vi "Feedback Message Loop.vi"(8 "error in (no error)":errorcluster, 10 "Data Notifiers":T2, 11 "Message Queues":T6) -> (0 "error out":errorcluster)   [LabVIEW 2013, in "Feedback.lvlib"]
uses:
  Feedback.lvlib
  support/Message Queue/All Message Queues.ctl
  support/Message Queue/Message Cluster.ctl
  Feedback State.ctl
  Feedback Parameters.ctl
  Scan Parameters.ctl
  support/Data Notifiers/All Data Notifiers.ctl
  Acquisition/APD Notifier Cluster.ctl
  Piezo/Piezo display.ctl
  XY/XY Display.ctl
  Capacitive/Capacitive Signal Cluster.ctl
  Error Signal.ctl
  piezo new/Hardware Configuration Piezo.ctl
  <vilib>/Utility/error.llb/Error Cluster From Error Code.vi
  support/Message Queue/Enqueue Message (Single).vi
  <vilib>/ErrorRing/Error Ring.xnode
  support/Message Queue/Message Queue.lvlib
  Piezo/Piezo.lvlib
  Acquisition/Acquisition.lvlib
  XY/XY.lvlib
  support/Data Notifiers/Data Notifiers.lvlib
  Capacitive/Capacitive.lvlib
panel:
  in  "Feedback Settings 2":T1={"Setpoint (cnt)"=3.0, "Refresh Time (s)"=1.0, "K_p (nm/cnt)"=0.01, "Averaging Time"=1.0, "T_i (s)"=1.0, "T_d (s)"=0.0, "Error Signal Source"=0} {"Error Signal Source" items=["External Input", "APD Signal"]}
  in  "Feedback Settings":T1={"Setpoint (cnt)"=3.0, "Refresh Time (s)"=1.0, "K_p (nm/cnt)"=0.01, "Averaging Time"=1.0, "T_i (s)"=1.0, "T_d (s)"=0.0, "Error Signal Source"=0} {"Error Signal Source" items=["External Input", "APD Signal"]}
  out "running average":dbl[](graph)
  out "Feedback State":T3 {"Feedback Parameters"."Error Signal Source" items=["External Input", "APD Signal"]}
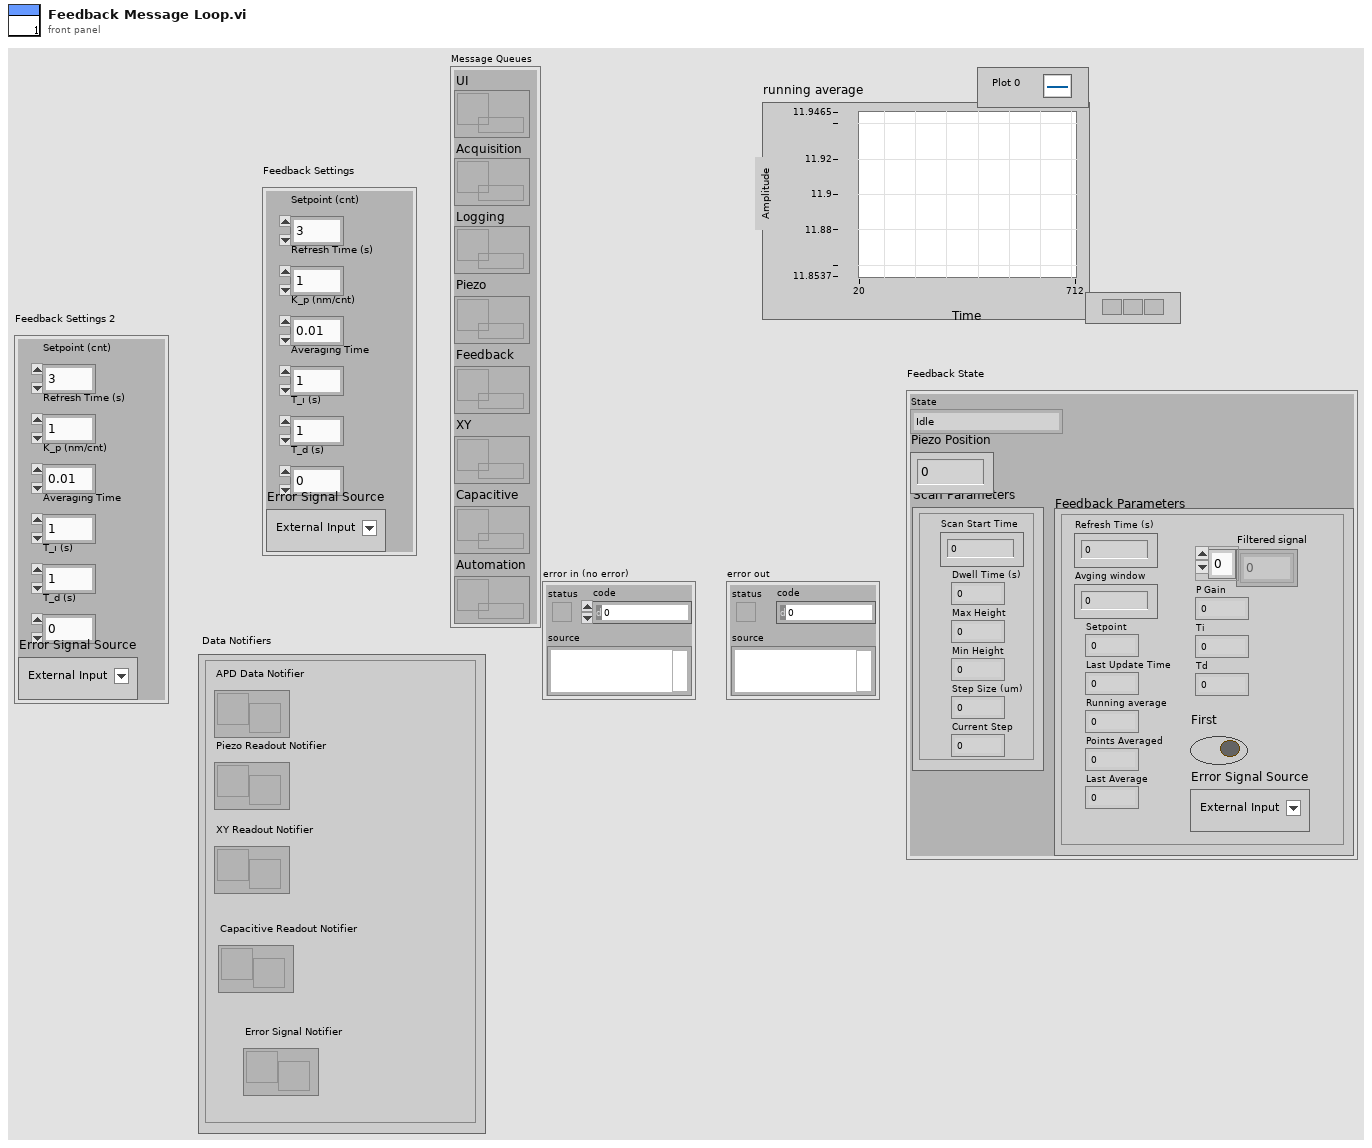
[diagram p1: front panel]
types:
  T1 = cluster{"Setpoint (cnt)":dbl, "Refresh Time (s)":dbl, "K_p (nm/cnt)":dbl, "Averaging Time":dbl, "T_i (s)":dbl, "T_d (s)":dbl, "Error Signal Source":u16}
  T2 = typedef "Data Notifiers.lvlib/All Data Notifiers.ctl" = cluster{"APD Data Notifier":refnum<notifier>, "Piezo Readout Notifier":refnum<notifier>, "XY Readout Notifier":refnum<notifier>, "Capacitive Readout Notifier":refnum<notifier>, "Error Signal Notifier":refnum<notifier>}
  T3 = typedef "Feedback.lvlib/Feedback State.ctl" = cluster{"State":enum16{"Idle", "Feedback", "Scanning", "Averaging"}, "Feedback Parameters":T4, "Scan Parameters":T5, "Piezo Position":dbl}
  T4 = typedef "Feedback.lvlib/Feedback Parameters.ctl" = cluster{"Refresh Time (s)":dbl, "P Gain":dbl, "Setpoint":dbl, "Last Update Time":dbl, "Running average":dbl, "Points Averaged":dbl, "Last Average":dbl, "Filtered signal":dbl[], "Avging window":dbl, "Ti":dbl, "Td":dbl, "First":bool, "Error Signal Source":u16}
  T5 = typedef "Feedback.lvlib/Scan Parameters.ctl" = cluster{"Scan Start Time":dbl, "Step Size (um)":dbl, "Min Height":dbl, "Max Height":dbl, "Dwell Time (s)":dbl, "Current Step":dbl}
  T6 = typedef "Message Queue.lvlib/All Message Queues.ctl" = cluster{"UI":refnum<queue>, "Acquisition":refnum<queue>, "Logging":refnum<queue>, "Piezo":refnum<queue>, "Feedback":refnum<queue>, "XY":refnum<queue>, "Capacitive":refnum<queue>, "Automation":refnum<queue>}
  T7 = typedef "Piezo.lvlib/Hardware Configuration Piezo.ctl" = cluster{"DAQmx Channel":tag, "Max Input":dbl, "Min Input":dbl, "Samples per ch.":dbl, "Setpoint (um)":dbl, "DAQmx Task":refnum<k21>}
  T8 = typedef "Feedback.lvlib/Error Signal.ctl" = cluster{"Error signal":dbl[], "Setpoint":dbl, "Last average":dbl}
  T9 = enum16{"Idle", "Feedback", "Scanning", "Averaging"}
  T10 = cluster{"Averaging Time (s)\n":dbl, "Error Signal Source":u16}
  T11 = cluster{"Dwell Time (s)":dbl, "Max Height":dbl, "Min Height":dbl, "Step Size (um)":dbl}
  T12 = typedef "Piezo.lvlib/Piezo display.ctl" = cluster{"PiezoPosition":sgl, "Counter Time":i32}
  T13 = typedef "Capacitive.lvlib/Capacitive Signal Cluster.ctl" = cluster{"Readout":sgl, "Time":i32, "Temperature":dbl}
  T14 = typedef "Acquisition.lvlib/APD Notifier Cluster.ctl" = cluster{"data":dbl[][], "t0":i32}
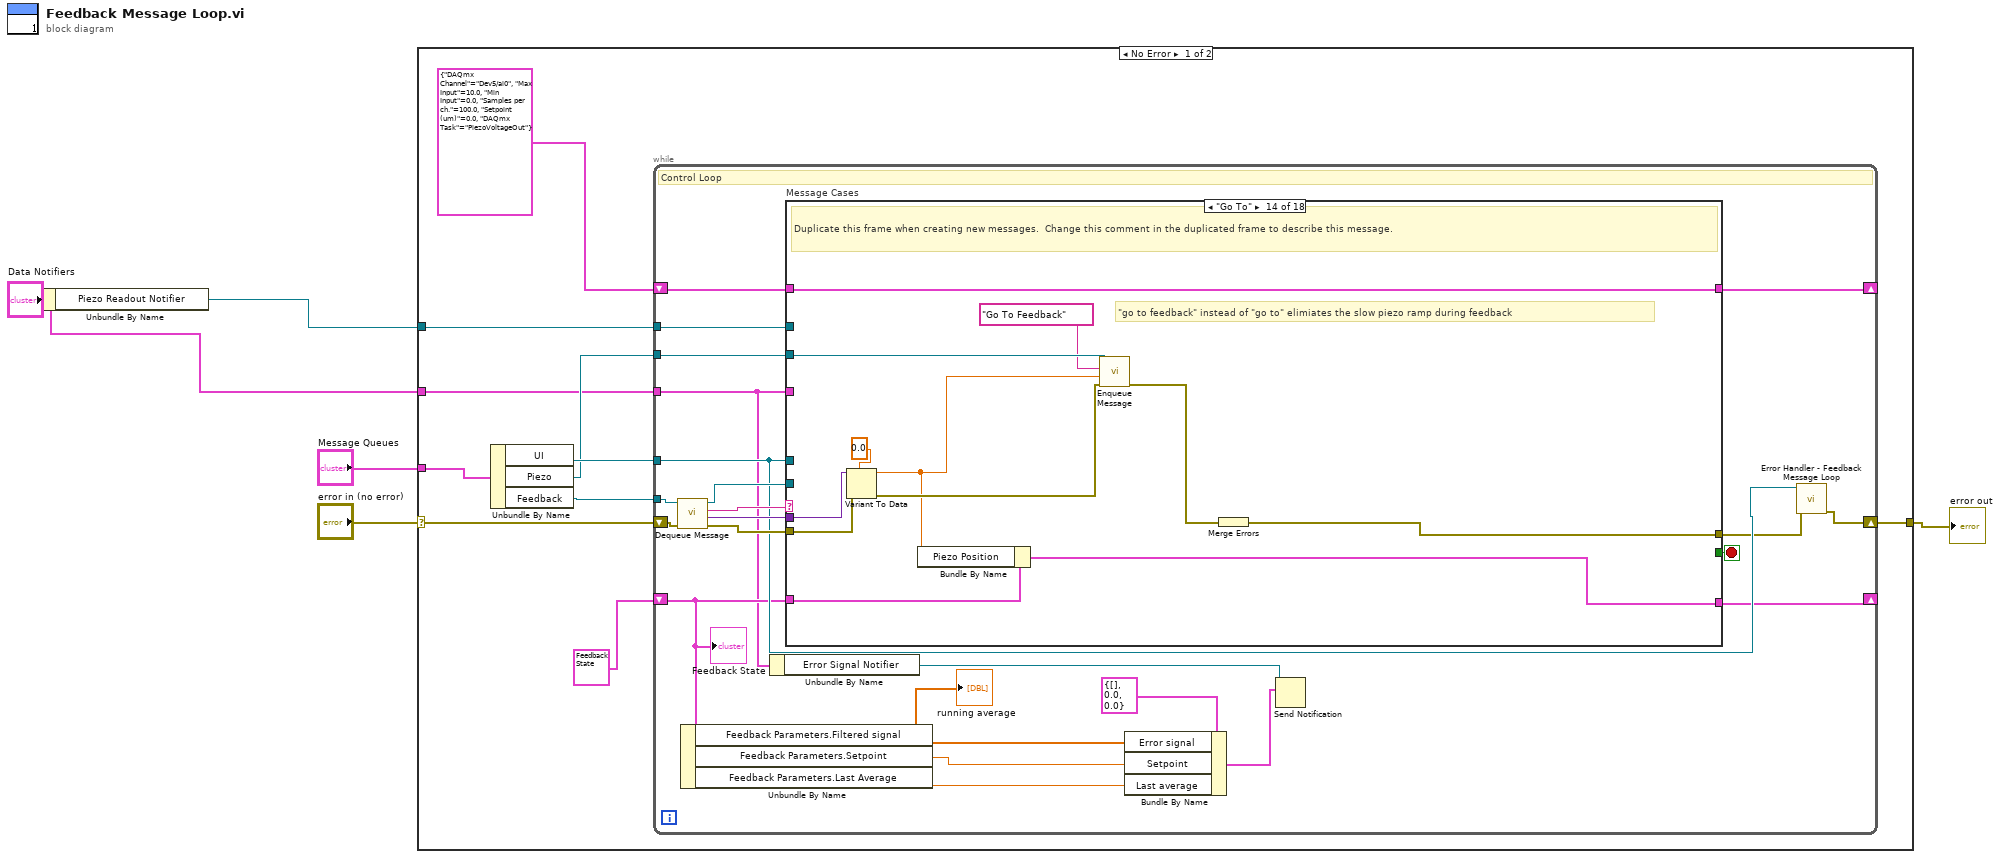
[diagram p0: block diagram]
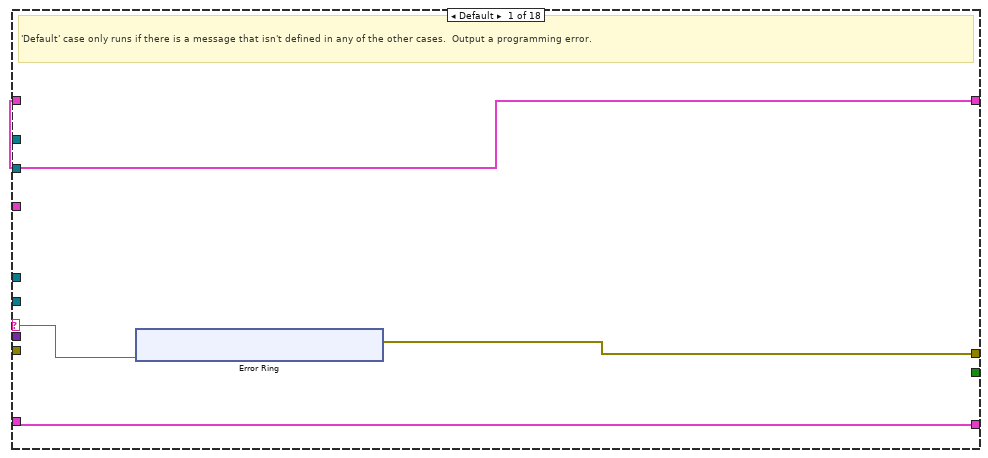
[diagram p2: hidden frame]
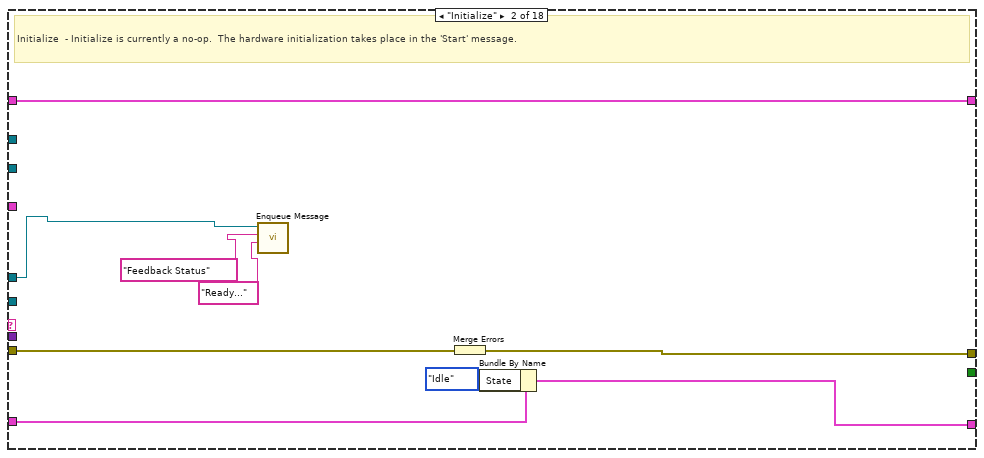
[diagram p3: hidden frame]
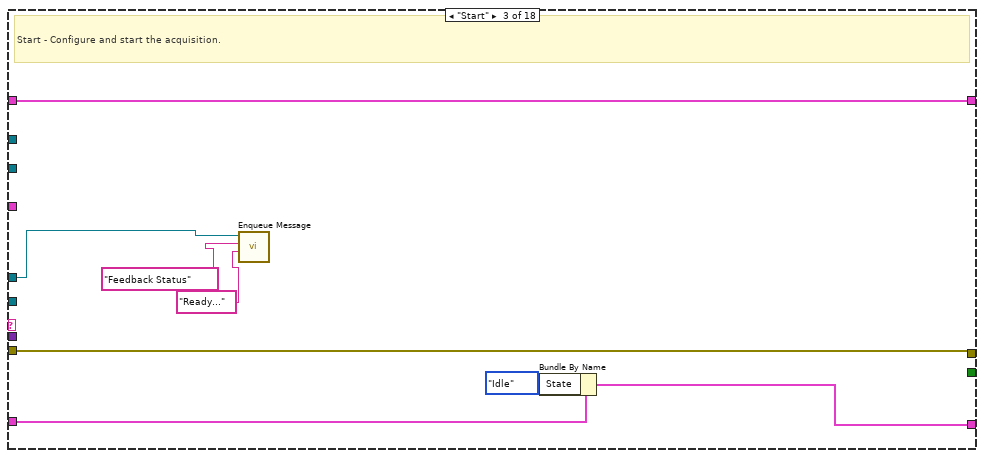
[diagram p4: hidden frame]
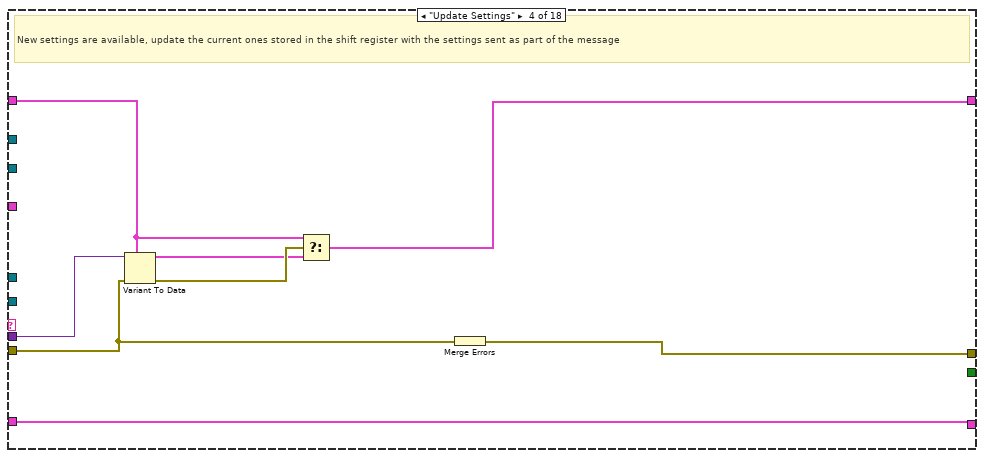
[diagram p5: hidden frame]
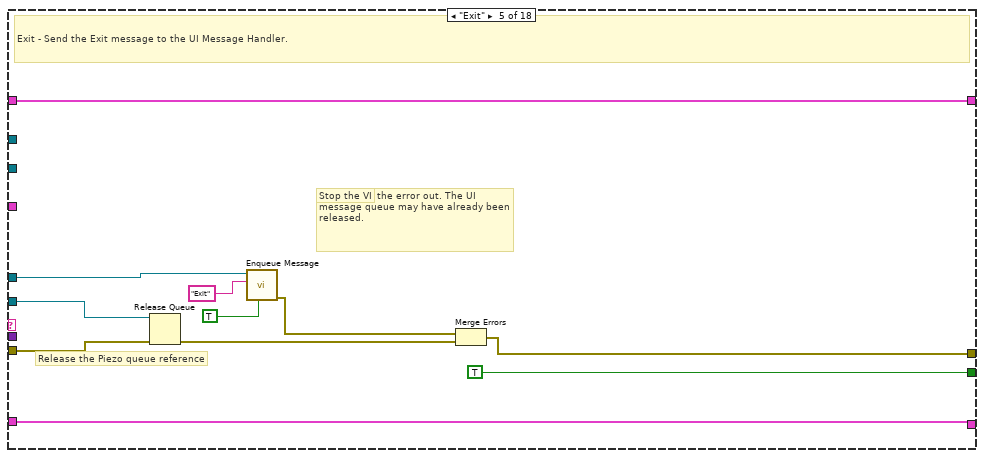
[diagram p6: hidden frame]
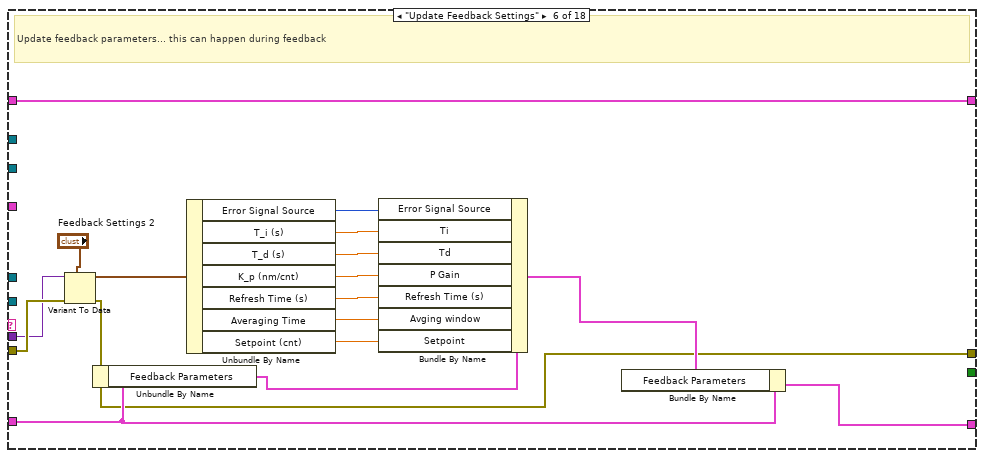
[diagram p7: hidden frame]
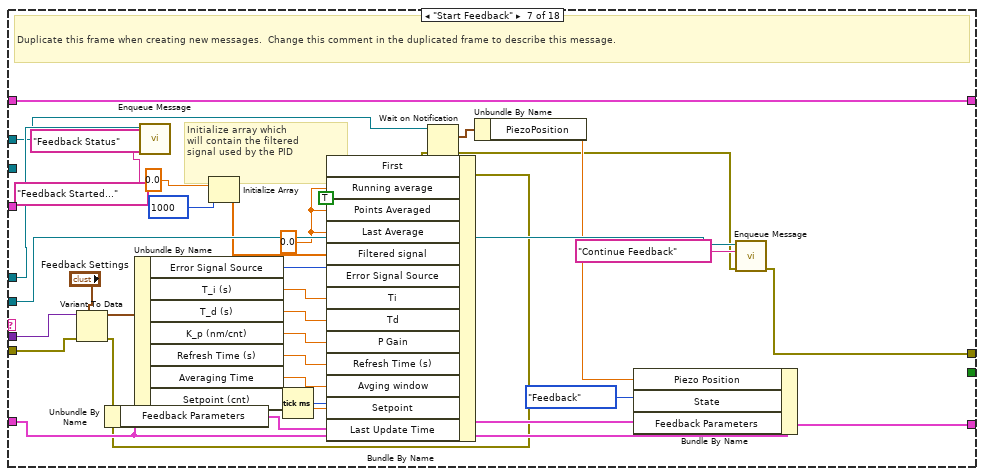
[diagram p8: hidden frame]
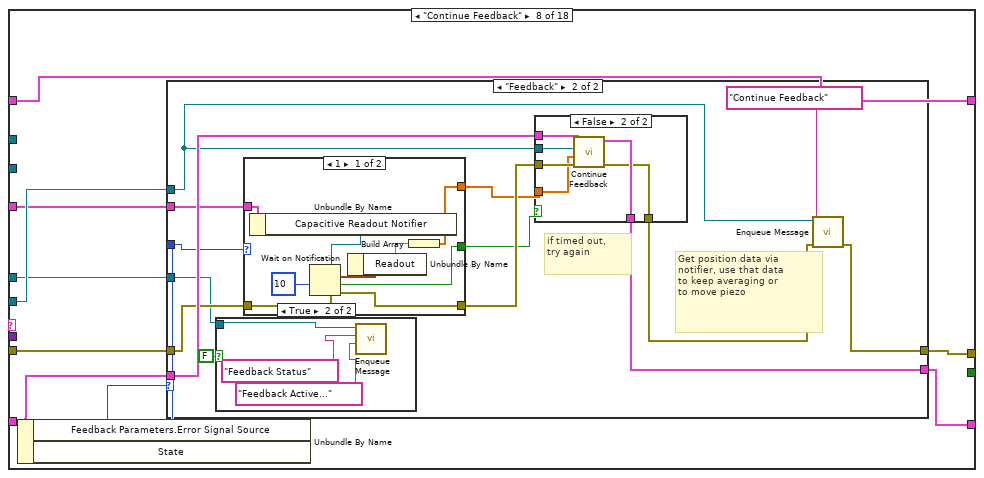
[diagram p9: hidden frame]
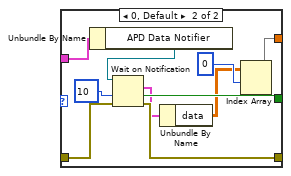
[diagram p12: hidden frame]
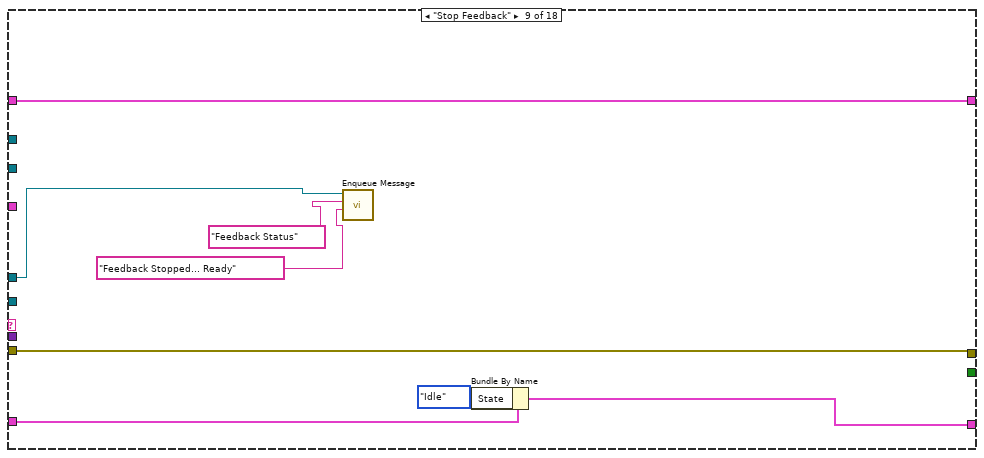
[diagram p14: hidden frame]
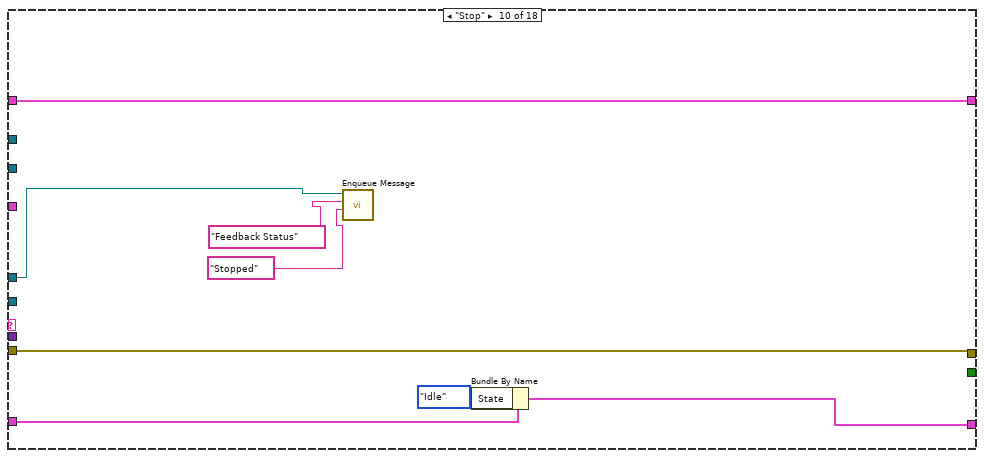
[diagram p15: hidden frame]
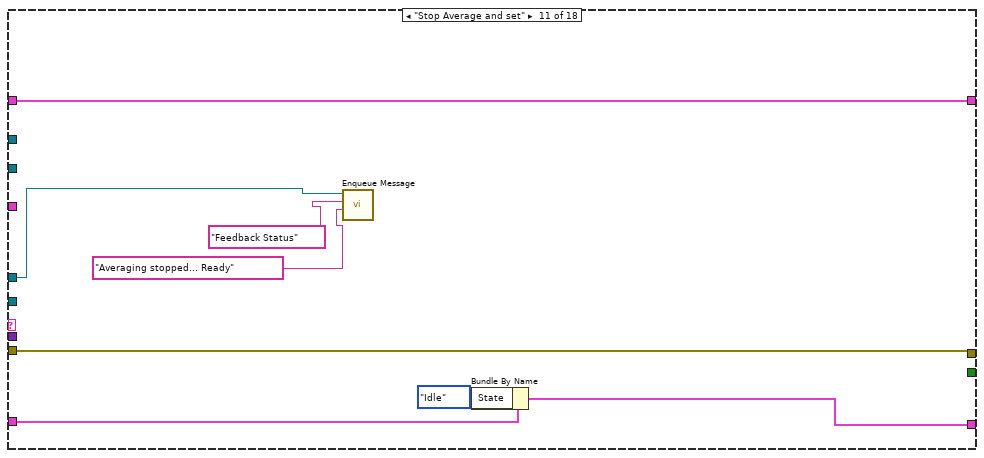
[diagram p16: hidden frame]
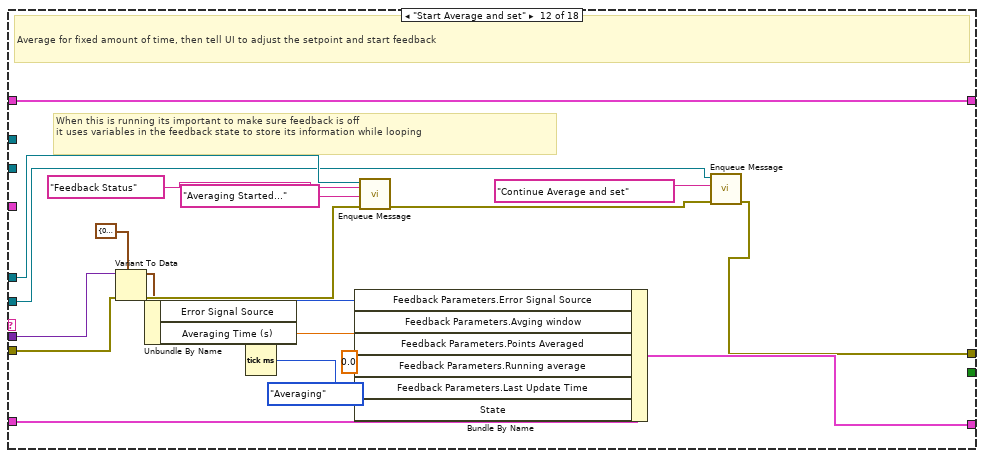
[diagram p17: hidden frame]
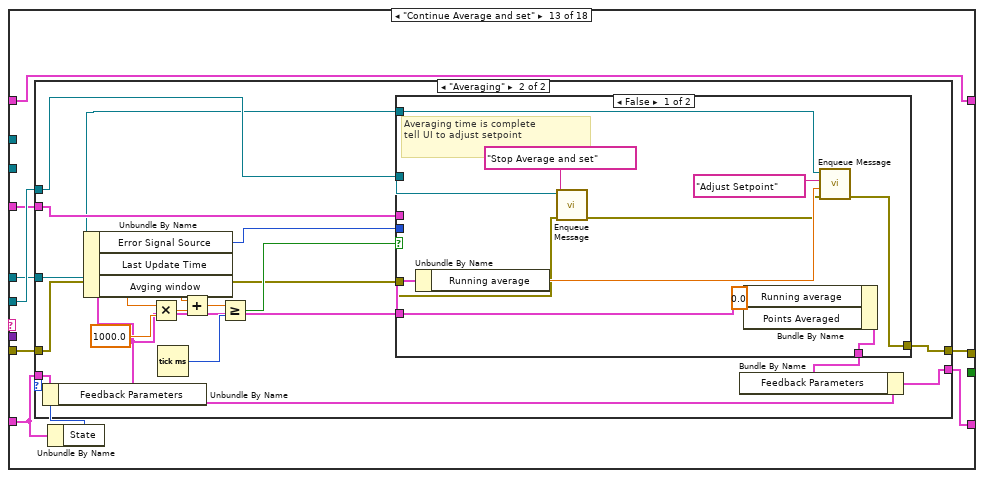
[diagram p18: hidden frame]
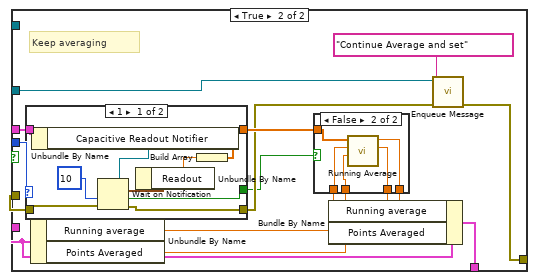
[diagram p20: hidden frame]
diagram:
  n1 = Unbundle By Name("Data Notifiers") -> ("Piezo Readout Notifier"=w2:refnum<notifier>)
  n2 = case shown="No Error" "error in (no error)" {
    selector: "error in (no error)" -> [w11 w389]
    tunnel: "Message Queues" -> [w15 _]
    tunnel: [w13 w389] -> w4
    tunnel: "Data Notifiers" -> [w9 _]
    tunnel: w2 -> [w8 _]
    frame No Error {
      n3 = Unbundle By Name(w15) -> ("UI"=w12:refnum<queue>, "Piezo"=w10:refnum<queue>, "Feedback"=w14:refnum<queue>)
      n4 = while {
        tunnel: w14 -> [w31]
        shift-right: [w30] -> _
        shift-left: T7 {"DAQmx Channel"="Dev5/ai0", "Max Input"=10.0, "Min Input"=0.0, "Samples per ch."=100.0, "Setpoint (um)"=0.0, "DAQmx Task"="PiezoVoltageOut"} ("Hardware Configuration") -> [w38]
        shift-right: [w27] -> w13
        shift-left: w11 -> [w36]
        tunnel: w12 -> [w29]
        tunnel: w10 -> [w26]
        tunnel: w9 -> [w22]
        tunnel: w8 -> [w25]
        shift-right: [w24] -> _
        shift-left: T3 {"State"=enum."Idle", "Feedback Parameters"={"Refresh Time (s)"=0.0, "P Gain"=0.0, "Setpoint"=0.0, "Last Update Time"=0.0, "Running average"=0.0, "Points Averaged"=0.0, "Last Average"=0.0, "Filtered signal"=[], "Avging window"=0.0, "Ti"=0.0, "Td"=0.0, "First"=FALSE, "Error Signal Source"=0}, "Scan Parameters"={"Scan Start Time"=0.0, "Step Size (um)"=0.0, "Min Height"=0.0, "Max Height"=0.0, "Dwell Time (s)"=0.0, "Current Step"=0.0}, "Piezo Position"=0.0} ("Feedback State") -> [w23]
        stop <- w37 stop-if-true
        # "Control Loop"
        n5 = call "Dequeue Message.vi"("error in (no error)"=w36, "Message Queue"=w31) -> ("error out"=w35:errorcluster, "Message Data"=w33:variant, "Message"=w34:string, "dup Message Queue"=w32:refnum<queue>)  [unwired: 6 in]
        n6 = Unbundle By Name(w23) -> ("Feedback Parameters.Filtered signal"=w16:dbl[], "Feedback Parameters.Setpoint"=w18:dbl, "Feedback Parameters.Last Average"=w17:dbl)
        "running average" <- w16
        n7 = Unbundle By Name(w22) -> ("Error Signal Notifier"=w21:refnum<notifier>)
        n8 = case "Message Cases" shown="\"Go To\"" w34 {
          selector: w34 -> [w42 _ _ _ _ _ _ _ _ _ _ _ _ _ _ _ _ _]
          tunnel: w32 -> [_ _ _ _ w81 _ w131 w140 _ _ _ w221 w239 _ w335 w361 _ _]
          tunnel: w35 -> [_ w57 w66 w69 w83 w89 w133 w145 w200 w208 w216 w232 w244 w325 w341 w359 w384 w388]
          tunnel: [w41 w58 w66 w74 w84 w88 w130 w144 w200 w208 w216 w223 w243 w328 w339 w354 w384 w387] -> w28
          tunnel: w38 -> [w40 w56 w65 w70 w80 w87 w136 w141 w196 w204 w212 w234 w240 w327 w336 w363 w383 w386]
          tunnel: [_ _ _ _ TRUE _ _ _ _ _ _ _ _ _ _ _ _ _] -> w37
          tunnel: w33 -> [_ _ _ w73 _ w86 w134 _ _ _ _ w233 _ w326 w345 _ _ _]
          tunnel: w29 -> [_ w53 w62 _ w77 _ w108 w138 w193 w201 w209 w225 w237 _ w329 w357 w377 _]
          tunnel: [w40 w56 w65 w68 w80 w87 w136 w141 w196 w204 w212 w234 w240 w327 w336 w363 w383 w386] -> w30
          tunnel: w26 -> [_ _ _ _ _ _ _ _ _ _ _ _ _ w323 _ _ _ _]
          tunnel: w22 -> [_ _ _ _ _ _ _ w139 _ _ _ _ w238 _ _ _ _ _]
          tunnel: w25 -> [_ _ _ _ _ _ w106 _ _ _ _ _ _ _ _ _ _ _]
          tunnel: w23 -> [w39 w51 w61 w67 w75 w91 w129 w142 w199 w207 w215 w236 w241 w319 w344 w360 w381 w385]
          tunnel: [w39 w50 w60 w67 w75 w90 w135 w143 w198 w206 w214 w235 w242 w318 w342 w358 w382 w385] -> w24
          frame Default {
            # "'Default' case only runs if there is a message that isn't defined in any of the other cases.  Output a programming error."
            n9 = xnode "Error Ring"("parameter 0"=w42) -> ("error out"=w41:errorcluster)
          }
          frame "Initialize" {
            # "Initialize  - Initialize is currently a no-op.  The hardware initialization takes place in the 'Start' message."
            n10 = call-poly "Enqueue Message.vi"("Message Data"="Ready..." ("Message"), "Message"="Feedback Status", "Message Queue"=w53) -> ()  [unwired: 7 in, 2 out]
            n11 = Merge Errors(w57) -> (w58:errorcluster)
            n12 = Bundle By Name(cluster=w51, "State"=T9."Idle") -> (w50:T3)
          }
          frame "Start" {
            # "Start - Configure and start the acquisition."
            n13 = call-poly "Enqueue Message.vi"("Message Data"="Ready..." ("Message"), "Message"="Feedback Status", "Message Queue"=w62) -> ()  [unwired: 7 in, 2 out]
            n14 = Bundle By Name(cluster=w61, "State"=T9."Idle") -> (w60:T3)
          }
          frame "Update Settings" {
            # "New settings are available, update the current ones stored in the shift register with the settings sent as part of the message"
            n15 = Variant To Data(error in=w69, type=w70, Variant=w73) -> (data=w71:T7, error out=w72:errorcluster)
            n16 = Select(t=w70, s=w72, f=w71) -> (s? t:f=w68:T7)
            n17 = Merge Errors(w69) -> (w74:errorcluster)
          }
          frame "Exit" {
            # "Don't check the error out. The UI message queue may have already been released."
            # "Release the Piezo queue reference"
            # "Stop the VI"
            # "Exit - Send the Exit message to the UI Message Handler."
            n18 = Release Queue(queue=w81, error in (no error)=w83) -> (error out=w82:errorcluster)  [unwired: 1 in, 2 out]
            n19 = call-poly "Enqueue Message.vi"("Priority Message? (F)"=TRUE, "Message"="Exit", "Message Queue"=w77) -> ("error out"=w76:errorcluster)  [unwired: 7 in, 1 out]
            n20 = Merge Errors(w76, w82) -> (w84:errorcluster)
          }
          frame "Update Feedback Settings" {
            # "Update feedback parameters... this can happen during feedback"
            n21 = Variant To Data(error in=w89, type="Feedback Settings 2", Variant=w86) -> (data=w100:T1, error out=w88:errorcluster)
            n22 = Unbundle By Name(w91) -> ("Feedback Parameters"=w101:T4)
            n23 = Unbundle By Name(w100) -> ("Error Signal Source"=w92:u16, "T_i (s)"=w94:dbl, "T_d (s)"=w93:dbl, "K_p (nm/cnt)"=w96:dbl, "Refresh Time (s)"=w99:dbl, "Averaging Time"=w98:dbl, "Setpoint (cnt)"=w97:dbl)
            n24 = Bundle By Name(cluster=w101, "Error Signal Source"=w92, "Ti"=w94, "Td"=w93, "P Gain"=w96, "Refresh Time (s)"=w99, "Avging window"=w98, "Setpoint"=w97) -> (w102:T4)
            n25 = Bundle By Name(cluster=w91, "Feedback Parameters"=w102) -> (w90:T3)
          }
          frame "Start Feedback" {
            w113 = 0.0 ("Last Average")
            # "Initialize array which\nwill contain the filtered \nsignal used by the PID"
            # "Duplicate this frame when creating new messages.  Change this comment in the duplicated frame to describe this message."
            n26 = Variant To Data(error in=w133, type="Feedback Settings", Variant=w134) -> (data=w124:T1, error out=w104:errorcluster)
            n27 = Unbundle By Name(w129) -> ("Feedback Parameters"=w125:T4)
            n28 = Unbundle By Name(w124) -> ("Error Signal Source"=w111:u16, "T_i (s)"=w115:dbl, "T_d (s)"=w114:dbl, "K_p (nm/cnt)"=w118:dbl, "Refresh Time (s)"=w123:dbl, "Averaging Time"=w122:dbl, "Setpoint (cnt)"=w121:dbl)
            n29 = call-poly "Enqueue Message.vi"("Message Data"="Feedback Started..." ("Message"), "Message"="Feedback Status", "Message Queue"=w108) -> ()  [unwired: 7 in, 2 out]
            n30 = Initialize Array(0.0 ("element"), 1000 ("dimension size")) -> (w117:dbl[])
            n31 = Tick Count (ms)() -> (millisecond timer value=w126:u32)
            n32 = Bundle By Name(cluster=w125, "First"=TRUE, "Running average"=w113, "Points Averaged"=w113, "Last Average"=w113, "Filtered signal"=w117, "Error Signal Source"=w111, "Ti"=w115, "Td"=w114, "P Gain"=w118, "Refresh Time (s)"=w123, "Avging window"=w122, "Setpoint"=w121, "Last Update Time"=w126) -> (w128:T4)
            n33 = Wait on Notification(notifier=w106, error in (no error)=w104) -> (notification=w107:T12, error out=w103:errorcluster)  [unwired: 2 in, 2 out]
            n34 = Unbundle By Name(w107) -> ("PiezoPosition"=w105:sgl)
            n35 = Bundle By Name(cluster=w129, "Piezo Position"=w105, "State"=enum16{"Idle", "Feedback", "Scanning"}."Feedback", "Feedback Parameters"=w128) -> (w135:T3)
            n36 = call-poly "Enqueue Message.vi"("error in (no error)"=w103, "Message"="Continue Feedback", "Message Queue"=w131) -> ("error out"=w130:errorcluster)  [unwired: 7 in, 1 out]
          }
          frame "Continue Feedback" {
            n37 = Unbundle By Name(w142) -> ("Feedback Parameters.Error Signal Source"=w137:u16, "State"=w146:T9)
            n38 = case shown="\"Feedback\"" w146 {
              tunnel: [w147 w154] -> w144
              tunnel: w145 -> [w147 w159]
              tunnel: [w148 w161] -> w143
              tunnel: w142 -> [w148 w162]
              tunnel: w140 -> [_ w156]
              tunnel: w139 -> [_ w152]
              tunnel: w138 -> [_ w151]
              tunnel: w137 -> [_ w149]
              frame "Idle", Default {
              }
              frame "Feedback" {
                # "if timed out,\ntry again"
                # "Get position data via\nnotifier, use that data\nto keep averaging or\nto move piezo"
                n39 = case shown="True" FALSE {
                  tunnel: w151 -> [_ w163]
                  frame False {
                  }
                  frame True {
                    n40 = call-poly "Enqueue Message.vi"("Message Data"="Feedback Active..." ("Message"), "Message"="Feedback Status", "Message Queue"=w163) -> ()  [unwired: 7 in, 2 out]
                  }
                }
                n41 = case shown="1" w149 {
                  tunnel: [w168 w184] -> w160
                  tunnel: w159 -> [w169 w183]
                  tunnel: [w170 w181] -> w158
                  tunnel: [w166 w175] -> w153
                  tunnel: w152 -> [w171 w179]
                  frame 1 {
                    n42 = Unbundle By Name(w171) -> ("Capacitive Readout Notifier"=w174:refnum<notifier>)
                    n43 = Wait on Notification(notifier=w174, timeout in ms (-1)=10, error in (no error)=w169) -> (notification=w173:T13, timed out?=w170:bool, error out=w168:errorcluster)  [unwired: 1 in, 1 out]
                    n44 = Unbundle By Name(w173) -> ("Readout"=w167:sgl)
                    n45 = Build Array(w167) -> (w166:sgl[])
                  }
                  frame 0, Default {
                    n46 = Unbundle By Name(w179) -> ("APD Data Notifier"=w178:refnum<notifier>)
                    n47 = Wait on Notification(notifier=w178, timeout in ms (-1)=10, error in (no error)=w183) -> (notification=w180:T14, timed out?=w181:bool, error out=w184:errorcluster)  [unwired: 1 in, 1 out]
                    n48 = Unbundle By Name(w180) -> ("data"=w176:dbl[][])
                    n49 = Index Array(array=w176, index (row)=0) -> (element=w175:dbl[])  [unwired: 1 in]
                  }
                }
                n50 = case shown="False" w158 {
                  tunnel: w162 -> [w186 w192]
                  tunnel: [w186 w191] -> w161
                  tunnel: [w185 w190] -> w155
                  tunnel: w156 -> [_ w189]
                  tunnel: w160 -> [w185 w188]
                  tunnel: w153 -> [_ w187]
                  frame True {
                  }
                  frame False {
                    n51 = call "Continue Feedback.vi"("error in (no error)"=w188, "notification"=w187, "Feedback Queue"=w189, "Feedback State In"=w192) -> ("error out"=w190:errorcluster, "Feedback State Out"=w191:T3)  [unwired: 4 in]
                  }
                }
                n52 = call-poly "Enqueue Message.vi"("error in (no error)"=w155, "Message"="Continue Feedback", "Message Queue"=w156) -> ("error out"=w154:errorcluster)  [unwired: 7 in, 1 out]
              }
            }
          }
          frame "Stop Feedback" {
            n53 = call-poly "Enqueue Message.vi"("Message Data"="Feedback Stopped... Ready" ("Message"), "Message"="Feedback Status", "Message Queue"=w193) -> ()  [unwired: 7 in, 2 out]
            n54 = Bundle By Name(cluster=w199, "State"=enum16{"Idle", "Feedback", "Scanning"}."Idle") -> (w198:T3)
          }
          frame "Stop" {
            n55 = call-poly "Enqueue Message.vi"("Message Data"="Stopped" ("Message"), "Message"="Feedback Status", "Message Queue"=w201) -> ()  [unwired: 7 in, 2 out]
            n56 = Bundle By Name(cluster=w207, "State"=enum16{"Idle", "Feedback", "Scanning"}."Idle") -> (w206:T3)
          }
          frame "Stop Average and set" {
            n57 = call-poly "Enqueue Message.vi"("Message Data"="Averaging stopped... Ready" ("Message"), "Message"="Feedback Status", "Message Queue"=w209) -> ()  [unwired: 7 in, 2 out]
            n58 = Bundle By Name(cluster=w215, "State"=enum16{"Idle", "Feedback", "Scanning"}."Idle") -> (w214:T3)
          }
          frame "Start Average and set" {
            w229 = 0.0 ("Feedback Parameters.Running average")
            # "When this is running its important to make sure feedback is off\nit uses variables in the feedback state to store its information while looping"
            # "Average for fixed amount of time, then tell UI to adjust the setpoint and start feedback"
            n59 = Variant To Data(error in=w232, type=T10 {"Averaging Time (s)\n"=0.0, "Error Signal Source"=0} ("output cluster"), Variant=w233) -> (data=w219:T10, error out=w226:errorcluster)
            n60 = Unbundle By Name(w219) -> ("Error Signal Source"=w217:u16, "Averaging Time (s)"=w218:dbl)
            n61 = Tick Count (ms)() -> (millisecond timer value=w230:u32)
            n62 = Bundle By Name(cluster=w236, "Feedback Parameters.Error Signal Source"=w217, "Feedback Parameters.Avging window"=w218, "Feedback Parameters.Points Averaged"=w229, "Feedback Parameters.Running average"=w229, "Feedback Parameters.Last Update Time"=w230, "State"=T9."Averaging") -> (w235:T3)
            n63 = call-poly "Enqueue Message.vi"("error in (no error)"=w226, "Message Data"="Averaging Started..." ("Message"), "Message"="Feedback Status", "Message Queue"=w225) -> ("error out"=w224:errorcluster)  [unwired: 6 in, 1 out]
            n64 = call-poly "Enqueue Message.vi"("error in (no error)"=w224, "Message"="Continue Average and set", "Message Queue"=w221) -> ("error out"=w223:errorcluster)  [unwired: 7 in, 1 out]
          }
          frame "Continue Average and set" {
            n65 = Unbundle By Name(w241) -> ("State"=w245:T9)
            n66 = case shown="\"Averaging\"" w245 {
              tunnel: [w246 w250] -> w243
              tunnel: w244 -> [w246 w251]
              tunnel: [w247 w252] -> w242
              tunnel: w241 -> [w247 w253]
              tunnel: w239 -> [_ w258]
              tunnel: w238 -> [_ w256]
              tunnel: w237 -> [_ w248]
              frame "Idle", Default {
              }
              frame "Averaging" {
                n67 = Unbundle By Name(w253) -> ("Feedback Parameters"=w255:T4)
                n68 = Unbundle By Name(w255) -> ("Error Signal Source"=w249:u16, "Last Update Time"=w261:dbl, "Avging window"=w264:dbl)
                n69 = Multiply(x=w264, y=1000.0) -> (x*y=w262:dbl)
                n70 = Tick Count (ms)() -> (millisecond timer value=w259:u32)
                n71 = Add(x=w261, y=w262) -> (x+y=w260:dbl)
                n72 = Greater Or Equal?(x=w260, y=w259) -> (x >= y?=w257:bool)
                n73 = case shown="False" w257 {
                  tunnel: w258 -> [w271 w289]
                  tunnel: w256 -> [_ w288]
                  tunnel: w255 -> [w270 w284]
                  tunnel: [w269 w281] -> w254
                  tunnel: w248 -> [w275 _]
                  tunnel: w251 -> [w267 w280]
                  tunnel: [w265 w278] -> w250
                  tunnel: w249 -> [_ w276]
                  frame False {
                    w268 = 0.0 ("Running average")
                    # "Averaging time is complete\ntell UI to adjust setpoint"
                    n74 = Unbundle By Name(w270) -> ("Running average"=w273:dbl)
                    n75 = call-poly "Enqueue Message.vi"("error in (no error)"=w267, "Message"="Stop Average and set", "Message Queue"=w271) -> ("error out"=w266:errorcluster)  [unwired: 7 in, 1 out]
                    n76 = Bundle By Name(cluster=w270, "Running average"=w268, "Points Averaged"=w268) -> (w269:T4)
                    n77 = call-poly "Enqueue Message.vi"("error in (no error)"=w266, "Message Data"=w273, "Message"="Adjust Setpoint", "Message Queue"=w275) -> ("error out"=w265:errorcluster)  [unwired: 6 in, 1 out]
                  }
                  frame True {
                    # "Keep averaging"
                    n78 = case shown="1" w276 {
                      tunnel: [w300 w316] -> w279
                      tunnel: w280 -> [w301 w315]
                      tunnel: [w302 w313] -> w277
                      tunnel: [w298 w307] -> w287
                      tunnel: w288 -> [w303 w311]
                      frame 1 {
                        n79 = Unbundle By Name(w303) -> ("Capacitive Readout Notifier"=w306:refnum<notifier>)
                        n80 = Wait on Notification(notifier=w306, timeout in ms (-1)=10, error in (no error)=w301) -> (notification=w305:T13, timed out?=w302:bool, error out=w300:errorcluster)  [unwired: 1 in, 1 out]
                        n81 = Unbundle By Name(w305) -> ("Readout"=w299:sgl)
                        n82 = Build Array(w299) -> (w298:sgl[])
                      }
                      frame 0, Default {
                        n83 = Unbundle By Name(w311) -> ("APD Data Notifier"=w310:refnum<notifier>)
                        n84 = Wait on Notification(notifier=w310, timeout in ms (-1)=10, error in (no error)=w315) -> (notification=w312:T14, timed out?=w313:bool, error out=w316:errorcluster)  [unwired: 1 in, 1 out]
                        n85 = Unbundle By Name(w312) -> ("data"=w309:dbl[][])
                        n86 = Index Array(array=w309, index (row)=0) -> (element=w307:dbl[])  [unwired: 1 in]
                      }
                    }
                    n87 = Unbundle By Name(w284) -> ("Running average"=w286:dbl, "Points Averaged"=w285:dbl)
                    n88 = case shown="False" w277 {
                      tunnel: w287 -> [_ w297]
                      tunnel: w286 -> [w291 w296]
                      tunnel: w285 -> [w292 w295]
                      tunnel: [w291 w294] -> w283
                      tunnel: [w292 w293] -> w282
                      frame True {
                      }
                      frame False {
                        n89 = call "Running Average.vi"("Points Averaged"=w295, "Running average"=w296, "notification"=w297) -> ("Points Avged Out"=w293:dbl, "Running Avg Out"=w294:dbl)  [unwired: 7 in]
                      }
                    }
                    n90 = Bundle By Name(cluster=w284, "Running average"=w283, "Points Averaged"=w282) -> (w281:T4)
                    n91 = call-poly "Enqueue Message.vi"("error in (no error)"=w279, "Message"="Continue Average and set", "Message Queue"=w289) -> ("error out"=w278:errorcluster)  [unwired: 7 in, 1 out]
                  }
                }
                n92 = Bundle By Name(cluster=w253, "Feedback Parameters"=w254) -> (w252:T3)
              }
            }
          }
          frame "Go To" {
            # "\"go to feedback\" instead of \"go to\" elimiates the slow piezo ramp during feedback"
            # "Duplicate this frame when creating new messages.  Change this comment in the duplicated frame to describe this message."
            n93 = Variant To Data(error in=w325, type=sgl 0.0, Variant=w326) -> (data=w317:sgl, error out=w321:errorcluster)
            n94 = Bundle By Name(cluster=w319, "Piezo Position"=w317) -> (w318:T3)
            n95 = call-poly "Enqueue Message.vi"("error in (no error)"=w321, "Message Data"=w317, "Message"="Go To Feedback", "Message Queue"=w323) -> ("error out"=w320:errorcluster)  [unwired: 6 in, 1 out]
            n96 = Merge Errors(w320) -> (w328:errorcluster)
          }
          frame "Start Scan" {
            # "Set to max height\nstart doing scan"
            n97 = Variant To Data(error in=w341, type=T11 {"Dwell Time (s)"=0.0, "Max Height"=0.0, "Min Height"=0.0, "Step Size (um)"=0.0}, Variant=w345) -> (data=w351:T11, error out=w333:errorcluster)
            n98 = Unbundle By Name(w351) -> ("Dwell Time (s)"=w350:dbl, "Max Height"=w338:dbl, "Min Height"=w349:dbl, "Step Size (um)"=w348:dbl)
            n99 = call-poly "Enqueue Message.vi"("Message Data"="Scan Started..." ("Message"), "Message"="Feedback Status", "Message Queue"=w329) -> ()  [unwired: 7 in, 2 out]
            n100 = Tick Count (ms)() -> (millisecond timer value=w353:u32)
            n101 = call-poly "Enqueue Message.vi"("error in (no error)"=w333, "Message Data"=w338, "Message"="Go To", "Message Queue"=w335) -> ("error out"=w332:errorcluster, "dup Message Queue"=w334:refnum<queue>)  [unwired: 6 in]
            n102 = Bundle By Name(cluster=w344, "Scan Parameters.Dwell Time (s)"=w350, "Scan Parameters.Max Height"=w338, "Scan Parameters.Min Height"=w349, "Scan Parameters.Step Size (um)"=w348, "Scan Parameters.Scan Start Time"=w353, "Scan Parameters.Current Step"=0.0 ("Current Step"), "State"=enum16{"Idle", "Feedback", "Scanning"}."Scanning") -> (w342:T3)
            n103 = call-poly "Enqueue Message.vi"("error in (no error)"=w332, "Message"="Continue Scan", "Message Queue"=w334) -> ("error out"=w340:errorcluster)  [unwired: 7 in, 1 out]
            n104 = Merge Errors(w340) -> (w339:errorcluster)
          }
          frame "Continue Scan" {
            # "If 'Stop' is called  from the UI, then the state switches to 'Idle'. Scanning only continues if State is 'Scanning'."
            n105 = Unbundle By Name(w360) -> ("State"=w362:T9)
            n106 = case shown="\"Scanning\"" w362 {
              tunnel: w361 -> [_ w376]
              tunnel: w360 -> [w371 w375]
              tunnel: w359 -> [w370 w374]
              tunnel: [w370 w373] -> w355
              tunnel: [w371 w372] -> w358
              frame "Idle", Default {
              }
              frame "Scanning" {
                n107 = call "Continue Scan.vi"("error in (no error)"=w374, "Feedback State In"=w375, "Feedback Queue"=w376) -> ("error out"=w373:errorcluster, "Feedback State Out"=w372:T3)  [unwired: 7 in]
              }
            }
            n108 = case shown="True" FALSE {
              tunnel: w357 -> [_ w367]
              tunnel: w355 -> [w364 w366]
              tunnel: [w364 w365] -> w354
              frame False {
              }
              frame True {
                n109 = call-poly "Enqueue Message.vi"("error in (no error)"=w366, "Message Data"="Scan In Progress..." ("Message"), "Message"="Feedback Status", "Message Queue"=w367) -> ("error out"=w365:errorcluster)  [unwired: 6 in, 1 out]
              }
            }
          }
          frame "Stop Scan" {
            n110 = call-poly "Enqueue Message.vi"("Message Data"="Scan Stopped... Ready" ("Message"), "Message"="Feedback Status", "Message Queue"=w377) -> ()  [unwired: 7 in, 2 out]
            n111 = Bundle By Name(cluster=w381, "State"=enum16{"Idle", "Feedback", "Scanning"}."Idle") -> (w382:T3)
          }
          frame "---Copy This Frame---" {
            # "Duplicate this frame when creating new messages.  Change this comment in the duplicated frame to describe this message."
            n112 = Merge Errors(w388) -> (w387:errorcluster)
          }
        }
        n113 = Bundle By Name(cluster=T8 {"Error signal"=[], "Setpoint"=0.0, "Last average"=0.0} ("Cluster"), "Error signal"=w16, "Setpoint"=w18, "Last average"=w17) -> (w19:T8)
        n114 = Send Notification(notification=w19, notifier=w21) -> ()  [unwired: 1 in, 2 out]
        n115 = call "Error Handler - Feedback Message Loop.vi"("error in (no error)"=w28, "Message Queue"=w29) -> ("dup error in"=w27:errorcluster)  [unwired: 8 in, 1 out]
        "Feedback State" <- w23
      }
    }
    frame Error {
    }
  }
  "error out" <- w4
